vi "FTW-TestExecutive-Core_LoadSequence.vi"(0 "FTW-TestExecutive-Core In":refnum<class "FTW-TestExecutive-Core.lvclass">, 5 "Sequence":string, 11 "error in":errorcluster) -> (4 "FTW-TestExecutive-Core Out":refnum<class "FTW-TestExecutive-Core.lvclass">, 8 "Loaded Sequence":T1[](array[typedef]) {"Results"."Start Time" format="%<%Y-%m-%d %H:%M:%S%03u>T"; "Results"."Elapsed Time" format="%<%H:%M:%S%3u>t"; "Elapsed Time" format="%<%H:%M:%S%3u>t"}, 15 "error out":errorcluster)   [LabVIEW 2018, in "FTW-TestExecutive-Core.lvclass"]
uses:
  FTW-TestExecutive-Core.lvclass
  FTW-TestExecutive-Step.ctl
  FTW-TestExecutive-Step-State.ctl
  FTW-TestExecutive-Results.ctl
  FTW-TestExecutive-Core.lvclass/FTW-TestExecutive-Core.ctl
  FTW-TestExecutive-Core_State.ctl
  JSON/FTW-JSON-JoinMode.ctl
  container/FTW-Container.lvclass
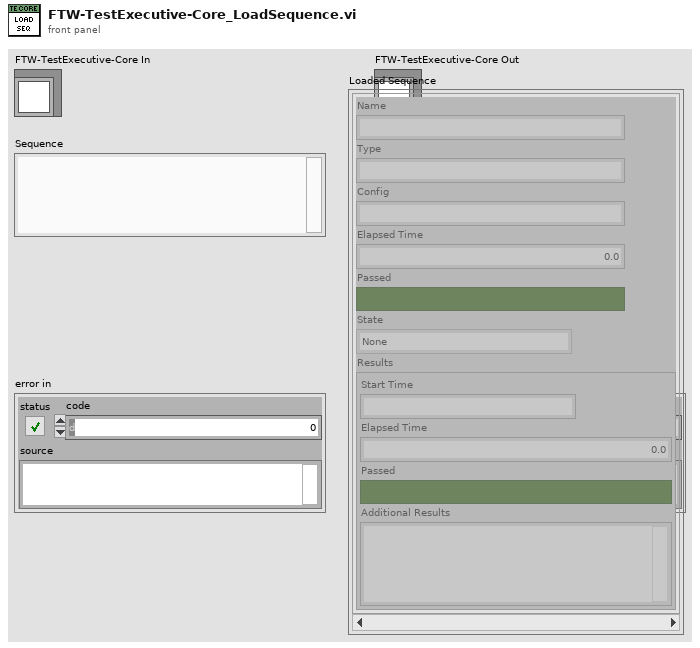
[diagram p1: front panel]
types:
  T1 = typedef "FTW-TestExecutive-Step.ctl" = cluster{"Name":string, "Type":string, "Config":string, "Elapsed Time":dbl, "Passed":bool, "State":T2, "Results":T3}
  T2 = typedef "FTW-TestExecutive-Step-State.ctl" = enum8{"None", "Failed", "Passed", "Timed out", "Aborted"}
  T3 = typedef "FTW-TestExecutive-Results.ctl" = cluster{"Start Time":timestamp, "Elapsed Time":dbl, "Passed":bool, "Additional Results":string}
  T4 = typedef "FTW-TestExecutive-Core.lvclass/FTW-TestExecutive-Core_State.ctl" = enum8{"Unloaded", "Loaded", "Executing", "Paused"}
  T5 = typedef "FTW-JSON-JoinMode.ctl" = enum32{"Upsert", "Update Only", "Insert Only"}
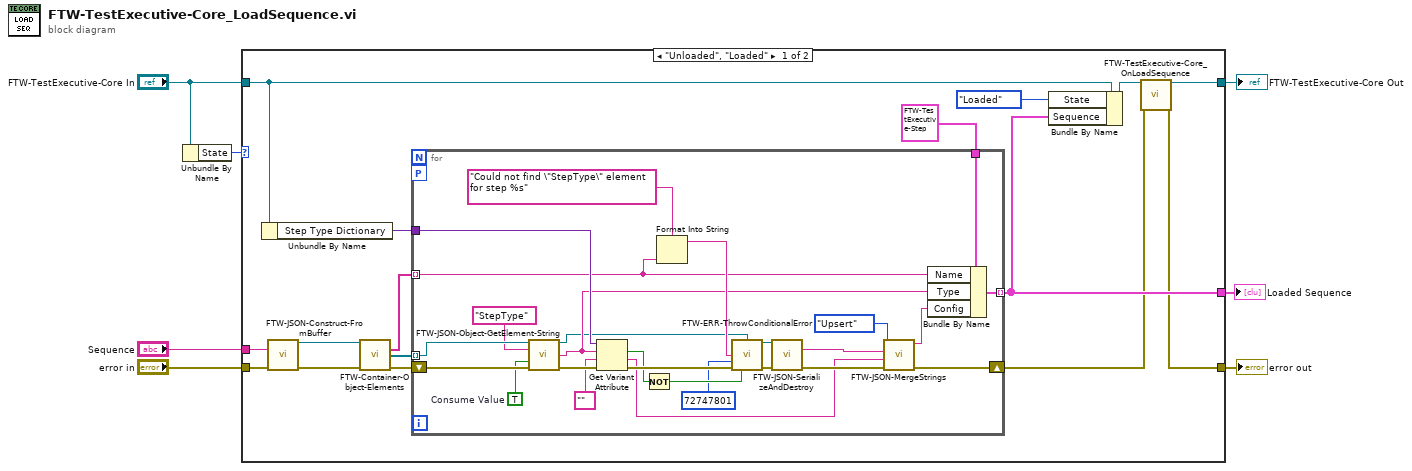
[diagram p0: block diagram]
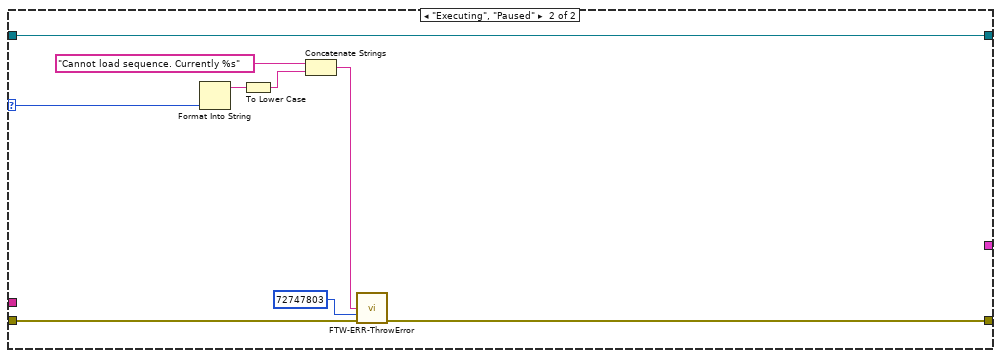
[diagram p2: hidden frame]
diagram:
  n1 = Unbundle By Name("FTW-TestExecutive-Core In") -> ("State"=w5:T4)
  n2 = case shown="\"Unloaded\", \"Loaded\"" w5 {
    selector: w5 -> [_ w53]
    tunnel: [w10 w57] -> w7
    tunnel: "FTW-TestExecutive-Core In" -> [w13 w57]
    tunnel: [w9 w55] -> w4
    tunnel: "error in" -> [w23 w56]
    tunnel: "Sequence" -> [w19 _]
    tunnel: [w11 _] -> w1
    frame "Unloaded", "Loaded" {
      n3 = Unbundle By Name(w13) -> ("Step Type Dictionary"=w16:variant)
      n4 = call "FTW-JSON-Construct-FromBuffer.vi"("JSON String (UTF-8)"=w19, "error in"=w23) -> ("JSON"=w18:refnum<class "FTW-Container.lvclass">, "error out"=w20:errorcluster)  [unwired: 12 in]
      n5 = call "FTW-Container-Object-Elements.vi"("FTW-Container In"=w18, "error in"=w20) -> ("Names"=w21:string[], "Object Elements"=w17:refnum<class "FTW-Container.lvclass">[], "error out"=w14:errorcluster)  [unwired: 10 in, 1 out]
      n6 = for {
        tunnel: w21 -> [w33] mode=indexing
        tunnel: w17 -> [w48] mode=indexing
        tunnel: w16 -> [w42]
        tunnel: [w32] -> w11 mode=indexing
        tunnel: T1 {"Name"="", "Type"="", "Config"="", "Elapsed Time"=0.0, "Passed"=FALSE, "State"=enum."None", "Results"={"Start Time"=timestamp(0 s since 1904-01-01), "Elapsed Time"=0.0, "Passed"=FALSE, "Additional Results"=""}} ("element") -> [w30]
        shift-right: [w28] -> w8
        shift-left: w14 -> [w47]
        workers-P: _ -> [_]
        w45 = TRUE  # Consume Value
        n7 = call "FTW-JSON-Object-GetElement-String.vi"("JSON"=w48, "Key"="StepType", "Consume Value"=w45, "error in"=w47) -> ("JSON out"=w29:refnum<class "FTW-Container.lvclass">, "Value"=w31:string, "error out"=w44:errorcluster)  [unwired: 7 in, 2 out]
        n8 = Get Variant Attribute(Variant=w42, name=w31, default value (empty Variant)="" ("empty string"), error in=w44) -> (found=w39:bool, value=w24:string, error out=w41:errorcluster)  [unwired: 1 out]
        n9 = Not(x=w39) -> (.not. x?=w38:bool)
        n10 = Format Into String(format string="Could not find \"StepType\" element for step %s" ("Error Message"), w33) -> (resulting string=w36:string)  [unwired: 2 in, 1 out]
        n11 = call "FTW-ERR-ThrowConditionalError.vi"("Error Message"=w36, "Error Code"=72747801, "error in"=w41, "Throw Error?"=w38) -> ("error out"=w40:errorcluster)  [unwired: 11 in]
        n12 = call "FTW-JSON-SerializeAndDestroy.vi"("JSON"=w29, "error in"=w40) -> ("JSON String (UTF-8)"=w25:string, "error out"=w34:errorcluster)  [unwired: 12 in]
        n13 = call "FTW-JSON-MergeStrings.vi"("error in (no error)"=w34, "Initial JSON String (\"\")"=w24, "JSON string to merge (\"\")"=w25, "Update Mode (0: Upsert)"=FTW-JSON-JoinMode."Upsert") -> ("error out"=w28:errorcluster, "Merged JSON String (UTF-8)"=w27:string)  [unwired: 6 in]
        n14 = Bundle By Name(cluster=w30, "Name"=w33, "Type"=w31, "Config"=w27) -> (w32:T1)
      }
      n15 = Bundle By Name(cluster=w13, "State"=FTW-TestExecutive-Core_State."Loaded", "Sequence"=w11) -> (w22:refnum<class "FTW-TestExecutive-Core.lvclass">)
      n16 = call "FTW-TestExecutive-Core_OnLoadSequence.vi"("FTW-TestExecutive-Core In"=w22, "error in"=w8) -> ("FTW-TestExecutive-Core Out"=w10:refnum<class "FTW-TestExecutive-Core.lvclass">, "error out"=w9:errorcluster)  [unwired: 12 in]
    }
    frame "Executing", "Paused" {
      n17 = Format Into String(w53) -> (resulting string=w52:string)  [unwired: 3 in, 1 out]
      n18 = To Lower Case(string=w52) -> (all lower case string=w50:string)
      n19 = Concatenate Strings("Cannot load sequence. Currently %s" ("Error Message"), w50) -> (w51:string)
      n20 = call "FTW-ERR-ThrowError.vi"("Error Message"=w51, "Error Code"=72747803, "error in"=w56) -> ("error out"=w55:errorcluster)  [unwired: 12 in]
    }
  }
  "FTW-TestExecutive-Core Out" <- w7
  "error out" <- w4
  "Loaded Sequence" <- w1
